vi "Create Subsystems.vi"(8 "error in (no error)":errorcluster, 9 "Subsystem I/O Attributes":T2[](array[typedef]), 10 "Subsystems":T1[](array[typedef]), 11 "System Name":string) -> (0 "error out":errorcluster)   [LabVIEW 2024]
doc: "Creates subsystems and I/O points of the subsystems in the shared variable engine."
uses:
  Controls/Server/Subsystem IO Attributes.ctl
  Controls/Server/Subsystem IO Logging Attributes.ctl
  Controls/Server/Subsystem IO Alarm Attributes.ctl
  Controls/Server/Subsystem Configuration.ctl
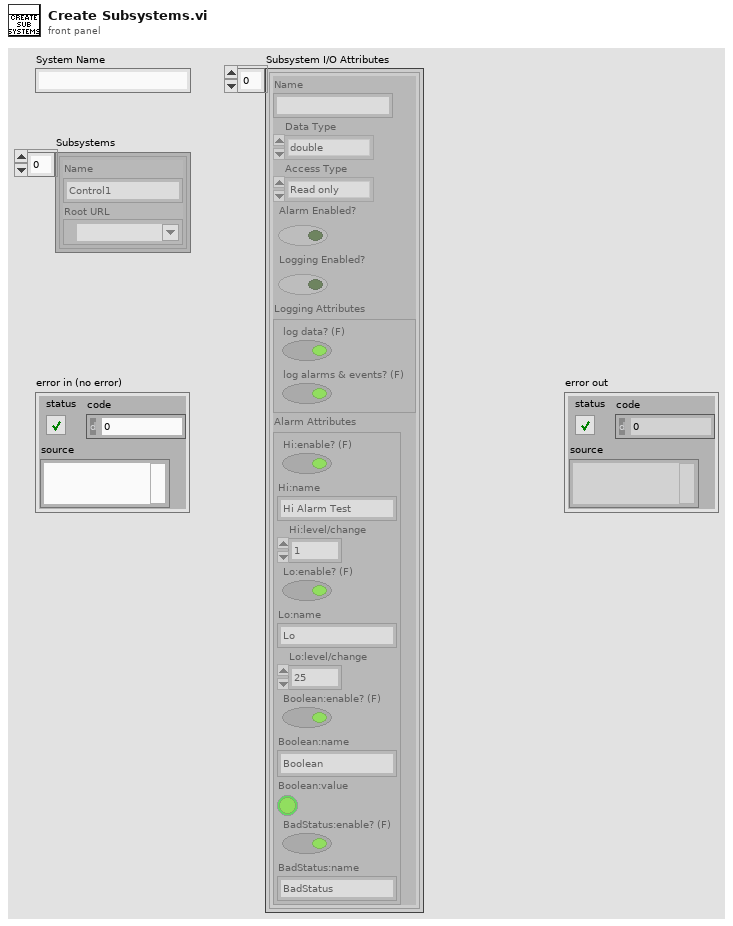
[diagram p1: front panel]
types:
  T1 = typedef "Subsystem Configuration.ctl" = cluster{"Name":string, "Root URL":refnum<k21>}
  T2 = typedef "Subsystem IO Attributes.ctl" = cluster{"Name":string, "Data Type":enum32{"u32BitField", "bool", "double", "string", "int8", "uint8", "int16", "uint16", "int32", "uint32", "int64", "uint64", "single", "double waveform", "int16 waveform", "array of boolean", "array of int8", "array of uint8", "array of int16", "array of uint16", "array of int32", "array of uint32", "array of int64", "array of uint64", "array of single", "array of double", "array of double waveform", "array of int16 waveform", "array of string", "variant", "timestamp", "fixed point", "custom"}, "Access Type":enum32{"Read only", "Write only", "Read/write"}, "Alarm Enabled?":bool, "Logging Enabled?":bool, "Logging Attributes":T3, "Alarm Attributes":T4}
  T3 = typedef "Subsystem IO Logging Attributes.ctl" = cluster{"log data? (F)":bool, "log alarms & events? (F)":bool}
  T4 = typedef "Subsystem IO Alarm Attributes.ctl" = cluster{"Hi:enable? (F)":bool, "Hi:name":string, "Hi:level/change":dbl, "Lo:enable? (F)":bool, "Lo:name":string, "Lo:level/change":dbl, "Boolean:enable? (F)":bool, "Boolean:name":string, "Boolean:value":bool, "BadStatus:enable? (F)":bool, "BadStatus:name":string}
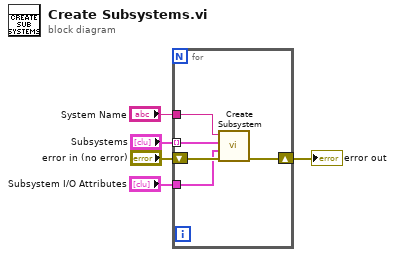
[diagram p0: block diagram]
diagram:
  n1 = for {
    shift-right: [w10] -> w3
    shift-left: "error in (no error)" -> [w9]
    tunnel: "Subsystems" -> [w7] mode=indexing
    tunnel: "Subsystem I/O Attributes" -> [w8]
    tunnel: "System Name" -> [w6]
    n2 = call "Create Subsystem.vi"("error in (no error)"=w9, "Subsystem I/O Attributes"=w8, "Subsystem"=w7, "System Name"=w6) -> ("error out"=w10:errorcluster)  [unwired: 7 in]
  }
  "error out" <- w3
